vi "averaged_stokes_acquisition_V2.vi"(0 "Motor \"Name\"":string="1", 2 "VISA resource name":refnum<visa-resource-name>="COM3", 5 "Encoder Pulses per Degree":i32=398, 7 "Number of Angles":i32=8, 9 "Number of Measures":i32=10, 11 "ICImagingControl In":refnum<k7>) -> (4 "Polarimetric Images 3D Array":dbl[][][](array[numeric]))   [LabVIEW 2025]
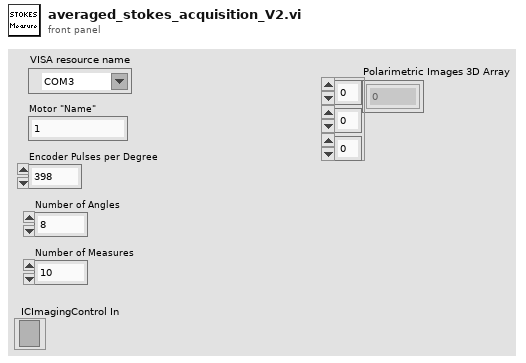
[diagram p1: front panel]
types:
  T1 = typedef "IMAQ Image.ctl" = refnum<image>
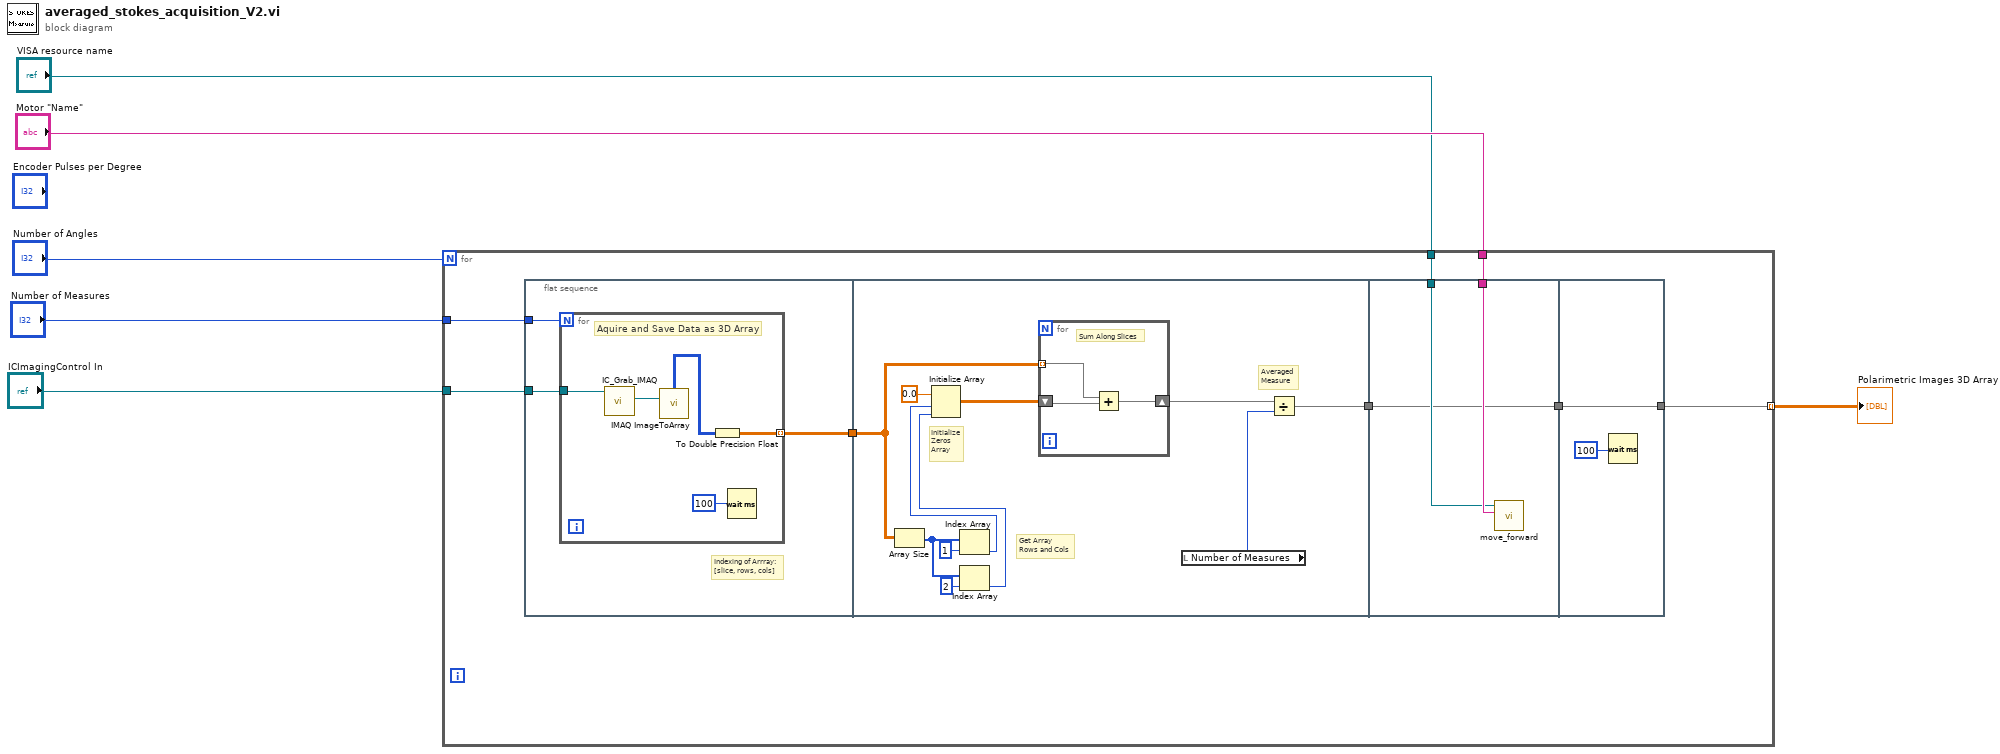
[diagram p0: block diagram]
diagram:
  n1 = for {
    N: "Number of Angles" -> [_]
    tunnel: "ICImagingControl In" -> [w14]
    tunnel: "Number of Measures" -> [w13]
    tunnel: "Motor \"Name\"" -> [w10]
    tunnel: "VISA resource name" -> [w9]
    tunnel: [w7] -> w1 mode=indexing
    n2 = flat-sequence {
      tunnel: w14 -> [w17]
      tunnel: w13 -> [w16]
      tunnel: [w15] -> w11
      tunnel: [w24] -> w12
      tunnel: w11 -> [w23]
      tunnel: w12 -> [w37]
      tunnel: w10 -> [w39]
      tunnel: w9 -> [w38]
      tunnel: [w37] -> w8
      tunnel: [w40] -> w7
      tunnel: w8 -> [w40]
      frame #0 {
        # "Indexing of Arrray:\n[slice, rows, cols]"
        n3 = for {
          N: w16 -> [_]
          tunnel: w17 -> [w21]
          tunnel: [w18] -> w15 mode=indexing
          # "Aquire and Save Data as 3D Array"
          n4 = call <userlib>:"IC_Grab_IMAQ.vi"("ICImagingControl In"=w21) -> ("Image Out"=w20:T1)  [unwired: 2 in, 3 out]
          n5 = call "IMAQ ImageToArray"("Image"=w20) -> ("Image Pixels (U8)"=w19:u8[][])  [unwired: 3 in, 4 out]
          n6 = To Double Precision Float(number=w19) -> (double precision float=w18:dbl[][])
          n7 = Wait (ms)(milliseconds to wait=u32 100) -> ()  [unwired: 1 out]
        }
      }
      frame #1 {
        # "Initialize\nZeros\nArray"
        # "Averaged\nMeasure"
        # "Get Array \nRows and Cols"
        n8 = Array Size(array=w23) -> (size(s)=w32:i32[])
        n9 = Index Array(array=w32, index=1) -> (element=w29:i32)
        n10 = Index Array(array=w32, index=2) -> (element=w28:i32)
        n11 = Initialize Array(0.0 ("element"), w29, w28) -> (w27:dbl[][])
        n12 = for {
          shift-right: [w35] -> w26
          shift-left: w27 -> [w36]
          tunnel: w23 -> [w34] mode=indexing
          # "Sum Along Slices"
          n13 = Add(x=w34, y=w36) -> (x+y=w35:dbl[][])
        }
        n14 = local read "Number of Measures"() -> (w25:i32)
        n15 = Divide(x=w26, y=w25) -> (x/y=w24:dbl[][])
      }
      frame #2 {
        n16 = call "move_forward.vi"("Motor \"Name\""=w39, "VISA resource name"=w38) -> ()  [unwired: 8 in, 2 out]
      }
      frame #3 {
        n17 = Wait (ms)(milliseconds to wait=u32 100) -> ()  [unwired: 1 out]
      }
    }
  }
  "Polarimetric Images 3D Array" <- w1
